vi "Send Event.vi"(5 "Tag Values":string[](array[string]), 6 "Event Type (info)":T1=enum."info", 7 "Tags":string[](array[string]), 8 "error in (no error)":errorcluster, 9 "Event Text":string, 10 "Event Title":string, 11 "StatD Interface in":refnum<class "StatD Interface.lvclass">) -> (0 "error out":errorcluster, 3 "StatD Interface out":refnum<class "StatD Interface.lvclass">)   [LabVIEW 2011, in "StatD Interface.lvclass"]
doc: "Sends an event to the statd collector."
uses:
  StatD Interface.lvclass
  Controls/Event Types.ctl
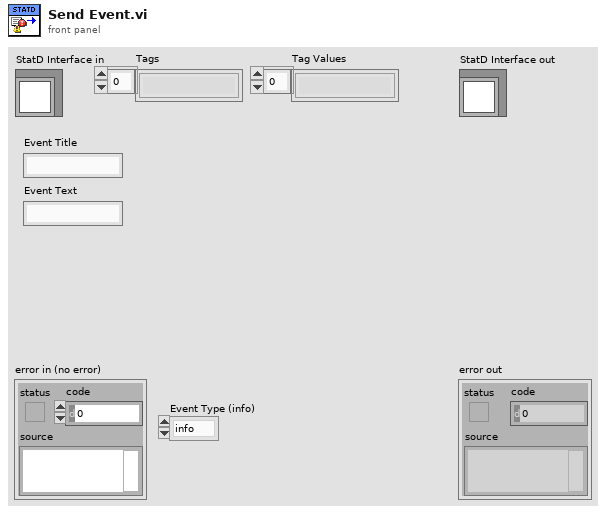
[diagram p1: front panel]
types:
  T1 = typedef "StatD Interface.lvclass/Event Types.ctl" = enum16{"error", "warning", "info", "success"}
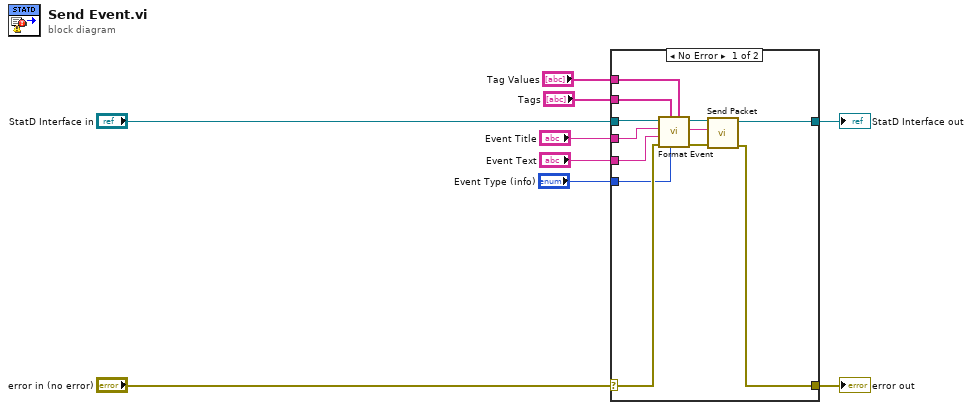
[diagram p0: block diagram]
diagram:
  n1 = case shown="No Error" "error in (no error)" {
    selector: "error in (no error)" -> [w15 w23]
    tunnel: [w18 w23] -> w8
    tunnel: [w19 w22] -> w6
    tunnel: "StatD Interface in" -> [w17 w22]
    tunnel: "Tags" -> [w14 _]
    tunnel: "Tag Values" -> [w13 _]
    tunnel: "Event Title" -> [w12 _]
    tunnel: "Event Text" -> [w11 _]
    tunnel: "Event Type (info)" -> [w10 _]
    frame No Error {
      n2 = call "Format Event.vi"("Tag Values"=w13, "Event Type"=w10, "Tags"=w14, "error in (no error)"=w15, "Event Text"=w11, "Event Title"=w12, "StatD Interface in"=w17) -> ("error out"=w16:errorcluster, "Packet"=w20:string, "StatD Interface out"=w21:refnum<class "StatD Interface.lvclass">)  [unwired: 2 in]
      n3 = call "Send Packet.vi"("error in (no error)"=w16, "Packet"=w20, "StatD Interface in"=w21) -> ("error out"=w18:errorcluster, "StatD Interface out"=w19:refnum<class "StatD Interface.lvclass">)  [unwired: 7 in]
    }
    frame Error {
    }
  }
  "error out" <- w8
  "StatD Interface out" <- w6
